vi "ShooterSpeedChoose.vi"(7 "Shooter OFF":bool, 9 "Close 3pt Shot Button":bool, 10 "Far 3pt Shot Button":bool, 11 "Feedershot Button":bool) -> (3 "Shooter Speed":T1(ring))   [LabVIEW 2012]
uses:
  Robot Global Data.vi
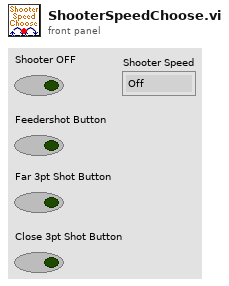
[diagram p1: front panel]
types:
  T1 = enum16{"Off", "Close Pyramid 3pt", "Far Pyramid 3pt", "Feeder Shot"}
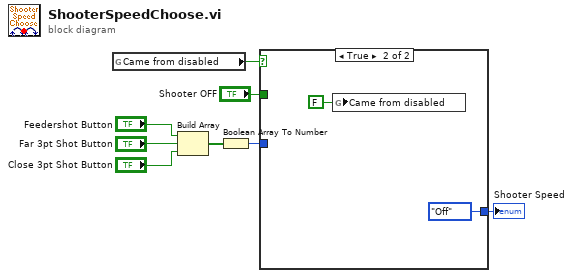
[diagram p0: block diagram]
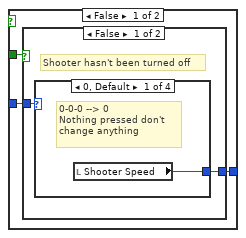
[diagram p2: hidden frame]
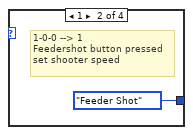
[diagram p3: hidden frame]
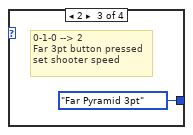
[diagram p4: hidden frame]
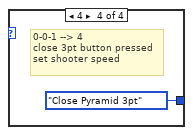
[diagram p5: hidden frame]
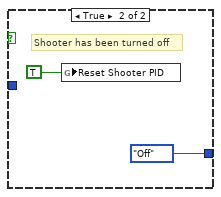
[diagram p6: hidden frame]
diagram:
  n1 = global read "Robot Global Data.vi" "Came from disabled"() -> (w1:bool)
  n2 = Build Array("Feedershot Button", "Far 3pt Shot Button", "Close 3pt Shot Button") -> (w8:bool[])
  n3 = Boolean Array To Number(Boolean array=w8) -> (number=w6:u32)
  n4 = case shown="True" w1 {
    tunnel: "Shooter OFF" -> [w11 _]
    tunnel: w6 -> [w10 _]
    tunnel: [w9 T1."Off" ("Shooter Speed")] -> w2
    frame False {
      n5 = case shown="False" w11 {
        tunnel: w10 -> [w13 _]
        tunnel: [w12 T1."Off" ("Shooter Speed")] -> w9
        frame False {
          # "Shooter hasn't been turned off"
          n6 = case shown="0, Default" w13 {
            tunnel: [w14 T1."Feeder Shot" ("Shooter Speed") T1."Far Pyramid 3pt" ("Shooter Speed") T1."Close Pyramid 3pt" ("Shooter Speed")] -> w12
            frame 0, Default {
              # "0-0-0 --> 0\nNothing pressed don't \nchange anything"
              n7 = local read "Shooter Speed"() -> (w14:T1)
            }
            frame 1 {
              # "1-0-0 --> 1\nFeedershot button pressed\nset shooter speed"
            }
            frame 2 {
              # "0-1-0 --> 2\nFar 3pt button pressed\nset shooter speed"
            }
            frame 4 {
              # "0-0-1 --> 4\nclose 3pt button pressed\nset shooter speed"
            }
          }
        }
        frame True {
          # "Shooter has been turned off"
          n8 = global write "Robot Global Data.vi" "Reset Shooter PID"(TRUE) -> ()
        }
      }
    }
    frame True {
      n9 = global write "Robot Global Data.vi" "Came from disabled"(FALSE ("Came from disabled")) -> ()
    }
  }
  "Shooter Speed" <- w2
